vi "fo_ExcelToDcm.vi"(6 "DICOM Info":path, 8 "error in (no error)":errorcluster, 10 "JournalPath":path, 11 "ServerInfo":T1={"port"=104, "AEtitle"="ME", "host"="127.0.0.1", "remoteAE"="STORESCP"}) -> (0 "error out":errorcluster, 3 "No active excel error":bool)   [LabVIEW 2013, in "main.lvlib"]
uses:
  main.lvlib
  Controls/Enum Variables.ctl
  C:/Users/Simon/SkyDrive/LabView/2013/DM2020/bin/Dicom.dll
  bin/Dicom.dll
  <userlib>/_OpenG.lib/file/file.llb/File Exists - Scalar__ogtk.vi
  <userlib>/_MGI/Error Handling/MGI Suppress Error Code/MGI Suppress Error Code (Scalar).vi
panel:
  in  "Excel._Worksheet":refnum<k7>
  in  "Excel._Application":refnum<k7>
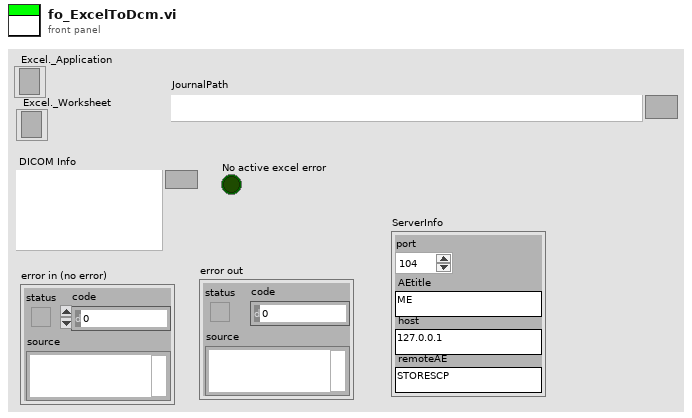
[diagram p1: front panel]
types:
  T1 = cluster{"port":i32, "AEtitle":string, "host":string, "remoteAE":string}
  T2 = typedef "main.lvlib/Enum Variables.ctl" = enum16{"SetAcqFilter", "GetAcqFilter", "Set Filter", "Get Filter", "Set Height", "Get Height", "Set Recorded Height", "Get Recorded Height", "Set Blue Pressure", "Get Blue Pressure", "Set Red Pressure", "Get Red Pressure", "Init", "Reset Pressure", "Set Red Cursors", "Get Red Cursors", "Set Blue Cursors", "Get Blue Cursors", "Set Language", "Get Language", "Set Active Graphs", "Get ActiveGraphs", "Set Method", "Get Method", "Set Encryption", "Get Encryption", "Set ExcelVersion", "Get ExcelVersion", "Set DICOM Avail", "Get DICOM Avail", "Set DICOM Encode", "Get DICOM Encode", "Set JournalExport", "Get JournalExport", "Set Sequence", "Get Sequence", "Set DAQ Connected", "Get DAQ Connected", "Set Current Graph", "Get Current Graph", "Set General Settings", "Get Hyphenation", "Set Arm Calc Method", "Get Arm Calc Method", "Set Dicom Tags", "Get Dicom Tags", "Set BT Serial", "Get BT Serial", "Set BT Accepted Serials", "Get BT Accepted Serials", "Get BT License", "Set BT License"}
  T3 = enum16{"leave excel open after last close", "close only if opened by LabVIEW", "close excel after last close"}
  T4 = enum16{"open workbook as template", "open workbook from file", "create new workbook"}
  T5 = typedef "excel Object Reference.ctl" = refnum<k1>
  T6 = typedef "excel Data Members.ctl" = cluster{"Excel._Application":refnum<k7>, "Excel._Workbook":refnum<k7>, "Excel._Worksheet":refnum<k7>, "template?":bool, "location":cluster{"TopLeft":string, "RightBottom":string}, "positioning info":cluster{"direction":enum16{"right", "down"}, "gap":i32}}
  T7 = cluster{"left":i16, "top":i16, "right":i16, "bottom":i16}
  T8 = cluster{"left":i32, "top":i32, "right":i32, "bottom":i32}
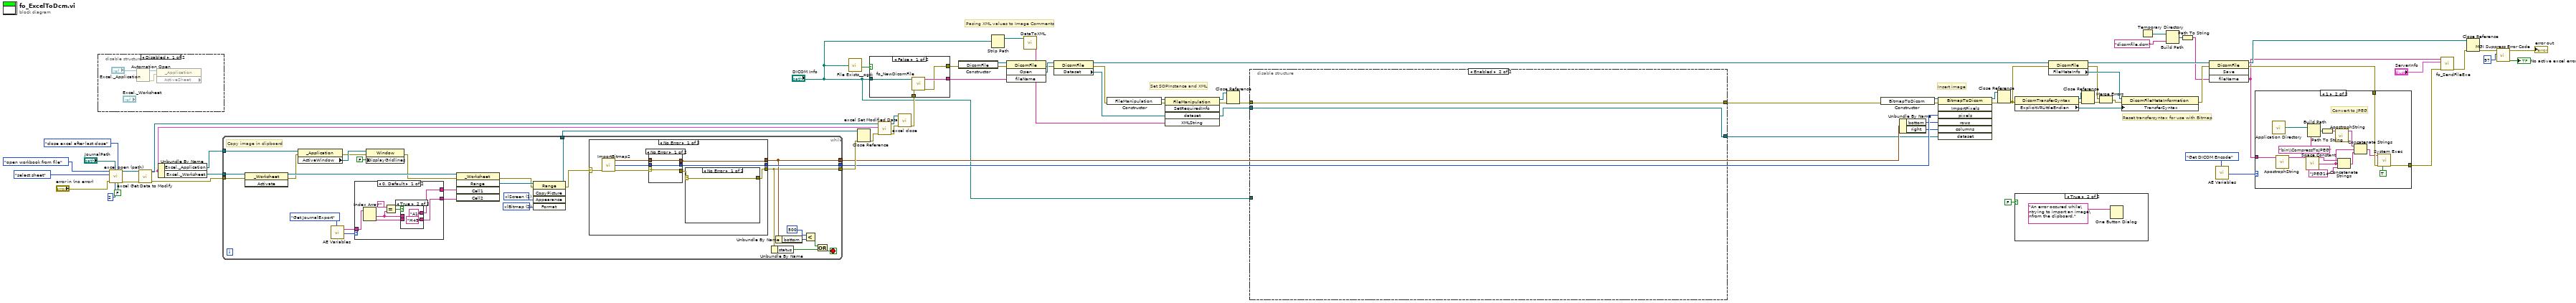
[diagram p0: block diagram]
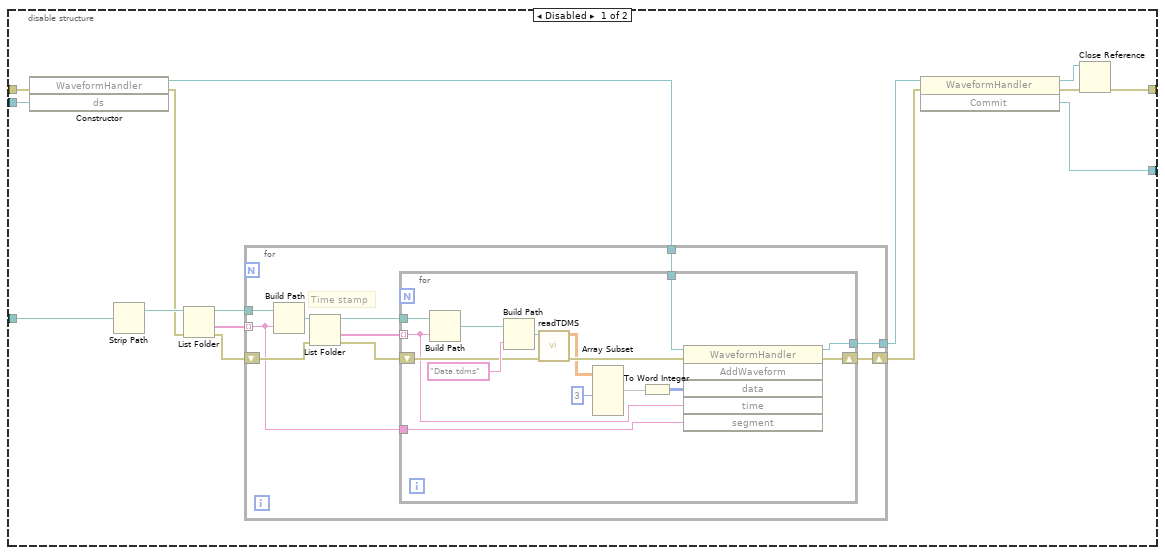
[diagram p2: hidden frame]
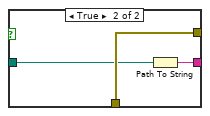
[diagram p4: hidden frame]
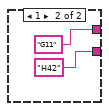
[diagram p8: hidden frame]
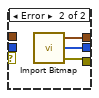
[diagram p9: hidden frame]
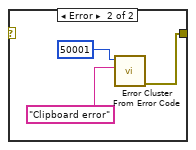
[diagram p10: hidden frame]
diagram:
  # "Reset transfersyntax for use with Bitmap"
  # "Set SOPInstance and XML"
  # "Insert image"
  # "Pasing XML values to Image Comments"
  n1 = disable-structure shown="Disabled" {
    frame Disabled {
      n2 = Automation Open(Automation Refnum="Excel._Application") -> (Automation Refnum=w76:refnum<k7>, error out=w75:errorcluster)  [unwired: 3 in]
      n3 = property class="_Application" props=["ActiveSheet"](reference=w76, error in=w75) -> ()  [unwired: 3 out]
    }
    frame Enabled {
    }
  }
  n4 = call <userlib>:"excel open (path).vi"("Visible (T)"=FALSE, "closing behavior (leave open)"=T3."close excel after last close", "worksheet_number"=u8 2, "workbook path"="JournalPath", "error in (no error)"="error in (no error)", "select/new"=enum16{"new sheet", "select sheet"}."select sheet", "create/open template/open file"=T4."open workbook from file") -> ("error out"=w64:errorcluster, "reference"=w65:T5)  [unwired: 3 in]
  n5 = call <userlib>:"excel Get Data to Modify.vi"("error in (no error)"=w64, "reference"=w65) -> ("error out"=w62:errorcluster, "data"=w57:T6, "duplicate reference"=w59:T5)  [unwired: 2 in, 1 out]
  n6 = Unbundle By Name(w57) -> ("Excel._Application"=w13:refnum<k7>, "Excel._Worksheet"=w63:refnum<k7>)
  n7 = while {
    tunnel: w62 -> [w83]
    tunnel: [w99] -> w49
    tunnel: [w94] -> w71
    tunnel: [w98] -> w48
    tunnel: [w95] -> w72
    tunnel: w63 -> [w84]
    tunnel: w13 -> [w87]
    stop <- w91 stop-if-true
    w103 = 2 items=["xlBitmap"=2, "xlPicture"=-4147] ("Format")
    w104 = 1 items=["xlPrinter"=2, "xlScreen"=1] ("Appearance")
    # "Copy image in clipboard"
    n8 = invoke class="_Worksheet" method="Activate"(reference=w84, error in=w83) -> (reference out=w82:refnum<k7>, error out=w81:errorcluster)  [unwired: 1 in, 1 out]
    n9 = property class="_Application"(reference=w87, error in=w81) -> (error out=w80:errorcluster, "ActiveWindow"=w86:refnum<k7>)  [unwired: 1 out]
    n10 = call "AE Variables.vi"("Action"=Enum_Variables."Get JournalExport") -> ("stringArray"=w78:string[], "RingOut"=w88:u16)  [unwired: 11 in, 6 out]
    n11 = case shown="0, Default" w88 {
      tunnel: [w107 "G11"] -> w102
      tunnel: [w106 "H42"] -> w101
      tunnel: w78 -> [w112 _]
      frame 0, Default {
        n12 = Index Array(array=w112) -> (element #1=w109:string, element #2=w108:string)  [unwired: 2 in]
        n13 = Equal?(x="", y=w109) -> (x = y?=w111:bool)
        n14 = case shown="True" w111 {
          tunnel: w109 -> [w114 _]
          tunnel: w108 -> [w113 _]
          tunnel: [w114 "A1"] -> w107
          tunnel: [w113 "H49"] -> w106
          frame False {
          }
          frame True {
          }
        }
      }
      frame 1 {
      }
    }
    n15 = property class="Window"(reference=w86, error in=w80, "DisplayGridlines"=FALSE) -> (error out=w79:errorcluster)  [unwired: 1 out]
    n16 = invoke class="_Worksheet" method="Range"(reference=w82, error in=w79, "Cell1"=w102, "Cell2"=w101) -> (error out=w100:errorcluster, "Range"=w105:refnum<k7>)  [unwired: 1 in, 3 out]
    n17 = invoke class="Range" method="CopyPicture"(reference=w105, error in=w100, "Appearance"=w104, "Format"=w103) -> (reference out=w95:refnum<k7>, error out=w90:errorcluster)  [unwired: 1 in, 3 out]
    n18 = case shown="No Error" w90 {
      selector: w90 -> [w119 w137]
      tunnel: [w125 _] -> w99
      tunnel: [w126 _] -> w98
      tunnel: [w123 w137] -> w94
      frame No Error {
        n19 = call "ImportBitmap2.vi"("error in (no error)"=w119) -> ("error out"=w120:errorcluster, "pixmap data"=w121:u8[], "rect"=w122:T7)  [unwired: 6 in, 2 out]
        n20 = case shown="No Error" w120 {
          selector: w120 -> [w127 _]
          tunnel: [w129 w132] -> w126
          tunnel: w122 -> [w129 _]
          tunnel: w121 -> [w128 _]
          tunnel: [w128 w131] -> w125
          tunnel: [w127 w130] -> w124
          frame No Error {
          }
          frame Error {
            n21 = call "Import Bitmap.vi"() -> ("rect"=w132:T8, "flattened data"=w131:u8[], "error out"=w130:errorcluster)  [unwired: 5 in, 2 out]
          }
        }
        n22 = case shown="No Error" w124 {
          selector: w124 -> [w133 _]
          tunnel: [w133 w136] -> w123
          frame No Error {
          }
          frame Error {
            n23 = call <vilib>:"Error Cluster From Error Code.vi"("error message (\"\")"="Clipboard error" ("error message (\"\")"), "error code (0)"=50001) -> ("error out"=w136:errorcluster)  [unwired: 7 in]
          }
        }
      }
      frame Error {
      }
    }
    n24 = Unbundle By Name(w94) -> ("status"=w92:bool)
    n25 = Unbundle By Name(w98) -> ("bottom"=w97:i32)
    n26 = Less?(x=500, y=w97) -> (x < y?=w93:bool)
    n27 = Or(x=w93, y=w92) -> (x .or. y?=w91:bool)
  }
  n28 = call-poly <userlib>:"File Exists__ogtk.vi"("file path"="DICOM Info") -> ("exists"=w30:bool)  [unwired: 6 in, 1 out]
  n29 = Close Reference(reference=w72, error in (no error)=w71) -> (error out=w61:errorcluster)
  n30 = call <userlib>:"excel Set Modified Data.vi"("error in (no error)"=w61, "data"=w57, "reference"=w59) -> ("error out"=w60:errorcluster, "duplicate reference"=w58:T5)  [unwired: 3 in]
  n31 = call <userlib>:"excel close.vi"("error in (no error)"=w60, "reference"=w58) -> ("error out"=w32:errorcluster)  [unwired: 9 in]
  n32 = case shown="False" w30 {
    tunnel: "DICOM Info" -> [w141 w142]
    tunnel: [w140 w143] -> w33
    tunnel: w32 -> [w139 w144]
    tunnel: [w138 w144] -> w31
    frame False {
      n33 = call "fo_NewDicomFile.vi"("error in (no error)"=w139, "DICOM Info"=w141) -> ("error out"=w138:errorcluster, "String"=w140:string)  [unwired: 8 in]
    }
    frame True {
      n34 = Path To String(path=w142) -> (string=w143:string)
    }
  }
  n35 = constructor class="DicomFile"(error in=w31) -> (reference out=w74:refnum<k24>, error out=w73:errorcluster)  [unwired: 2 in, 1 out]
  n36 = Strip Path(path="DICOM Info") -> (stripped path=w14:path)  [unwired: 1 out]
  n37 = invoke class="DicomFile" method="Open"(reference=w74, error in=w73, "fileName"=w33) -> (error out=w53:errorcluster, "Open"=w54:refnum<k24>)  [unwired: 1 in, 2 out]
  n38 = call "DataToXML.vi"("path"=w14) -> ("XML"=w28:string)  [unwired: 9 in, 1 out]
  n39 = property class="DicomFile"(reference=w54, error in=w53) -> (reference out=w22:refnum<k24>, error out=w24:errorcluster, "Dataset"=w7:refnum<k24>)
  n40 = constructor class="FileManipulation"(error in=w24) -> (reference out=w29:refnum<k24>, error out=w27:errorcluster)  [unwired: 2 in, 1 out]
  n41 = invoke class="FileManipulation" method="SetRequiredInfo"(reference=w29, error in=w27, "dataset"=w7, "XMLString"=w28) -> (reference out=w25:refnum<k24>, error out=w26:errorcluster)  [unwired: 1 in, 3 out]
  n42 = Close Reference(reference=w25, error in (no error)=w26) -> (error out=w8:errorcluster)
  n43 = disable-structure shown="Enabled" {
    disable-tunnel: w8 -> [w159 w186]
    disable-tunnel: w7 -> [w158 w185]
    disable-tunnel: [w157 w185] -> w6
    disable-tunnel: [w154 w186] -> w5
    disable-tunnel: "DICOM Info" -> [w153 _]
    frame Disabled {
      n44 = constructor class="WaveformHandler"(error in=w159, "ds"=w158) -> (reference out=w146:refnum<k24>, error out=w149:errorcluster)  [unwired: 2 in, 2 out]
      n45 = Strip Path(path=w153) -> (stripped path=w152:path)  [unwired: 1 out]
      n46 = List Folder(path=w152, error in=w149) -> (path out=w150:path, folder names=w151:string[], error out=w148:errorcluster)  [unwired: 2 in, 1 out]
      n47 = for {
        tunnel: w151 -> [w160] mode=indexing
        tunnel: w150 -> [w168]
        shift-right: [w163] -> w147
        shift-left: w148 -> [w165]
        tunnel: w146 -> [w162]
        tunnel: [w161] -> w145
        # "Time stamp"
        n48 = Build Path(base path=w168, name or relative path=w160) -> (appended path=w169:path)
        n49 = List Folder(path=w169, error in=w165) -> (path out=w167:path, folder names=w166:string[], error out=w164:errorcluster)  [unwired: 2 in, 1 out]
        n50 = for {
          tunnel: w167 -> [w182]
          tunnel: w166 -> [w172] mode=indexing
          shift-right: [w178] -> w163
          shift-left: w164 -> [w180]
          tunnel: w162 -> [w177]
          tunnel: [w176] -> w161
          tunnel: w160 -> [w171]
          n51 = Build Path(base path=w182, name or relative path=w172) -> (appended path=w181:path)
          n52 = Build Path(base path=w181, name or relative path="Data.tdms") -> (appended path=w183:path)
          n53 = call "readTDMS.vi"("error in (no error)"=w180, "Path Out"=w183) -> ("error out"=w179:errorcluster, "Array"=w175:dbl[][])  [unwired: 8 in]
          n54 = Array Subset(array=w175, length (row)=3 ("length")) -> (w173:dbl[][])  [unwired: 3 in]
          n55 = To Word Integer(number=w173) -> (16bit integer=w170:i16[][])
          n56 = invoke class="WaveformHandler" method="AddWaveform"(reference=w177, error in=w179, "data"=w170, "time"=w172, "segment"=w171) -> (reference out=w176:refnum<k24>, error out=w178:errorcluster)  [unwired: 1 in, 4 out]
        }
      }
      n57 = invoke class="WaveformHandler" method="Commit"(reference=w145, error in=w147) -> (reference out=w155:refnum<k24>, error out=w156:errorcluster, "Commit"=w157:refnum<k24>)  [unwired: 1 in]
      n58 = Close Reference(reference=w155, error in (no error)=w156) -> (error out=w154:errorcluster)
    }
    frame Enabled {
    }
  }
  n59 = constructor class="BitmapToDicom"(error in=w5) -> (reference out=w50:refnum<k24>, error out=w45:errorcluster)  [unwired: 2 in, 1 out]
  n60 = Unbundle By Name(w48) -> ("bottom"=w47:i32, "right"=w46:i32)
  n61 = invoke class="BitmapToDicom" method="ImportPixels"(reference=w50, error in=w45, "pixels"=w49, "rows"=w47, "columns"=w46, "dataset"=w6) -> (reference out=w43:refnum<k24>, error out=w44:errorcluster)  [unwired: 1 in, 5 out]
  n62 = Close Reference(reference=w43, error in (no error)=w44) -> (error out=w18:errorcluster)
  n63 = property class="DicomTransferSyntax"(error in=w18) -> (reference out=w16:refnum<k24>, error out=w17:errorcluster, "ExplicitVRLittleEndian"=w20:refnum<k24>)  [unwired: 1 in]
  n64 = case shown="True" FALSE {
    frame False {
    }
    frame True {
      n65 = One Button Dialog(message="An error occured while\ntrying to import an image\nfrom the clipboard.") -> ()  [unwired: 1 in, 1 out]
    }
  }
  n66 = property class="DicomFile"(reference=w22, error in=w18) -> (reference out=w21:refnum<k24>, error out=w2:errorcluster, "FileMetaInfo"=w23:refnum<k24>)
  n67 = Close Reference(reference=w16, error in (no error)=w17) -> (error out=w4:errorcluster)
  n68 = Merge Errors(w2, w4) -> (w3:errorcluster)
  n69 = property class="DicomFileMetaInformation"(reference=w23, error in=w3, "TransferSyntax"=w20) -> (error out=w19:errorcluster)  [unwired: 1 out]
  n70 = Temporary Directory() -> (w12:path)
  n71 = Build Path(base path=w12, name or relative path="dicomfile.dcm") -> (appended path=w10:path)
  n72 = Path To String(path=w10) -> (string=w9:string)
  n73 = invoke class="DicomFile" method="Save"(reference=w21, error in=w19, "fileName"=w9) -> (reference out=w37:refnum<k24>, error out=w35:errorcluster)  [unwired: 1 in, 2 out]
  n74 = call "AE Variables.vi"("Action"=Enum_Variables."Get DICOM Encode") -> ("RingOut"=w15:u16)  [unwired: 11 in, 7 out]
  n75 = case shown="1" w15 {
    tunnel: w35 -> [w188 w202]
    tunnel: [w188 w201] -> w34
    tunnel: w9 -> [_ w199]
    frame 0, Default {
    }
    frame 1 {
      # "Convert to JPEG"
      n76 = call <vilib>:"Application Directory.vi"() -> ("Application Directory"=w196:path)
      n77 = call "ApostrophString.vi"("String in"=w199) -> ("String out"=w200:string)  [unwired: 10 in]
      n78 = call <vilib>:"Space Constant.vi"() -> ("String"=w190:string)
      n79 = Build Path(base path=w196, name or relative path="bin\\CompressToJPEG") -> (appended path=w194:path)
      n80 = Path To String(path=w194) -> (string=w193:string)
      n81 = call "ApostrophString.vi"("String in"=w193) -> ("String out"=w191:string)  [unwired: 10 in]
      n82 = Concatenate Strings(w200, w190, "JPEG14") -> (w192:string)
      n83 = Concatenate Strings(w191, w190, w192) -> (w189:string)
      n84 = call <vilib>:"System Exec.vi"("run minimized? (F)"=TRUE, "error in (no error)"=w202, "command line"=w189) -> ("error out"=w201:errorcluster)  [unwired: 5 in, 3 out]
    }
  }
  n85 = call "fo_SendFileExe.vi"("error in (no error)"=w34, "ServerInfo"="ServerInfo", "File"=w9) -> ("error out"=w38:errorcluster)  [unwired: 8 in]
  n86 = Close Reference(reference=w37, error in (no error)=w38) -> (error out=w36:errorcluster)
  n87 = call-poly <userlib>:"MGI Suppress Error Code.vi"("Error Code"=97, "Error In"=w36) -> ("Error Supressed?"=→"No active excel error":bool, "Error Out"=→"error out":errorcluster)  [unwired: 4 in]
